vi "WriteICP.vi"(8 "error in (no error)":errorcluster, 10 "ICP":bool, 11 "DataVer3 in":refnum<class "DataVer3.lvclass">) -> (0 "error out":errorcluster, 3 "DataVer3 out":refnum<class "DataVer3.lvclass">)   [LabVIEW 2013, in "DataVer3.lvclass"]
uses:
  DataVer3.lvclass
  DataVer3.lvclass/DataVer3.ctl
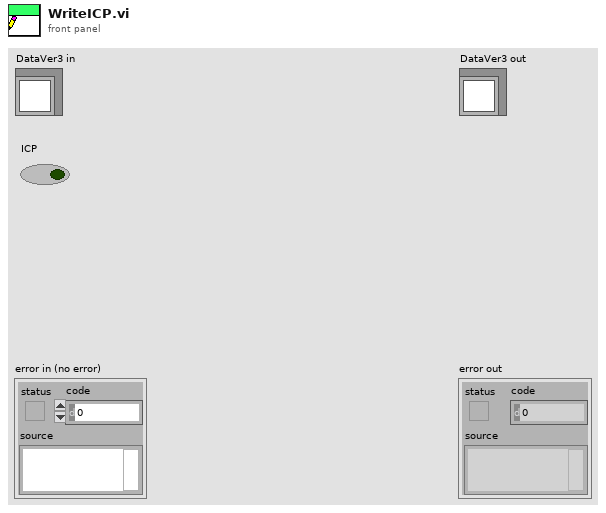
[diagram p1: front panel]
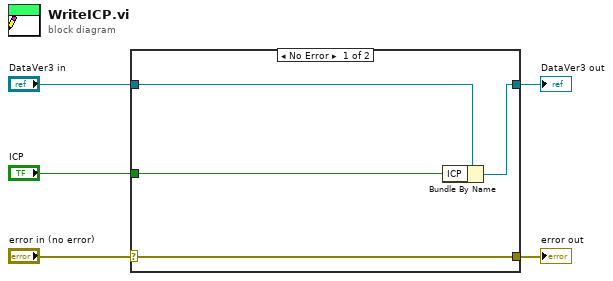
[diagram p0: block diagram]
diagram:
  n1 = case shown="No Error" "error in (no error)" {
    selector: "error in (no error)" -> [w9 w10]
    tunnel: [w9 w10] -> w4
    tunnel: [w7 w11] -> w2
    tunnel: "DataVer3 in" -> [w8 w11]
    tunnel: "ICP" -> [w6 _]
    frame No Error {
      n2 = Bundle By Name(cluster=w8, "ICP"=w6) -> (w7:refnum<class "DataVer3.lvclass">)
    }
    frame Error {
    }
  }
  "error out" <- w4
  "DataVer3 out" <- w2
